vi "Affichage PokaenDex.vi"() -> ()   [LabVIEW 2013]
uses:
  <vilib>/picture/picture.llb/Draw True-Color Pixmap.vi
panel:
  in  "Bouton OK 2":bool
  in  "Port USB en réception":refnum<visa-resource-name>="ASRL1::INSTR"
  out "Cache rouge":picture
  out "Ami 2":bool
  out "2":bool
  out "Image 2D":picture
  out "sign 2":u32
  out "Distance cible 2":string
  out "sign 1":u32
  out "Distance cible 1":string
  out "Cam D détect":bool
  out "2 cam détect":bool
  out "Cam G détect":bool
  in  "2D/3D":bool caption="Booléen 5"
  in  "Booléen":bool
  out "1":bool
  out "Ami":bool
  out "Cache gris":picture
  out "Nom du Pokaenmon":string
  out "Nom du Pokaenmon 2":string
  out "Pokeanmon détécté !":bool
  in  "stop":bool
  out "Image Pokaenmon 2":picture
  out "Image Pokaenmon":picture
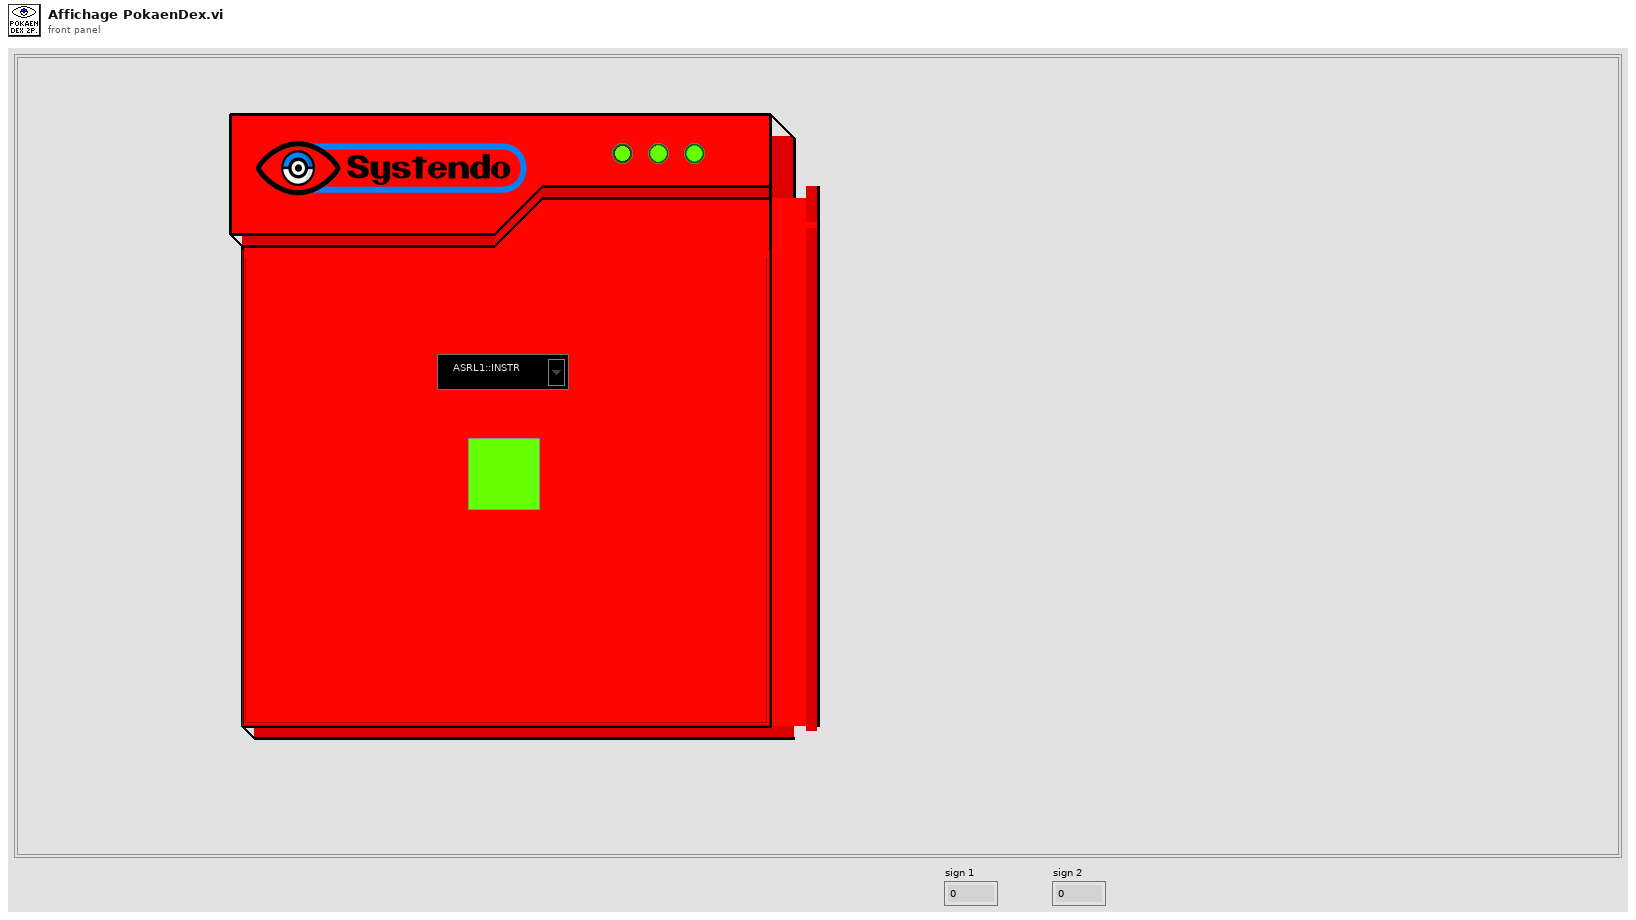
[diagram p1: front panel]
types:
  T1 = cluster{"left":i16, "top":i16, "right":i16, "bottom":i16}
  T2 = cluster{"Pokaenmon détecté":bool, "Signature":u32, "x":dbl, "y ":dbl, "Longueur":dbl, "Hauteur":dbl}
  T3 = cluster{"Données Caméra G":cluster{dbl, dbl, dbl, dbl}, "Données Caméra D":cluster{dbl, dbl, dbl, dbl}}
  T4 = typedef "imagedata.ctl" = cluster{"image type":i32, "image depth":i32, "image":u8[], "mask":u8[], "colors":u32[], "Rectangle":cluster{"left":i16, "top":i16, "right":i16, "bottom":i16}}
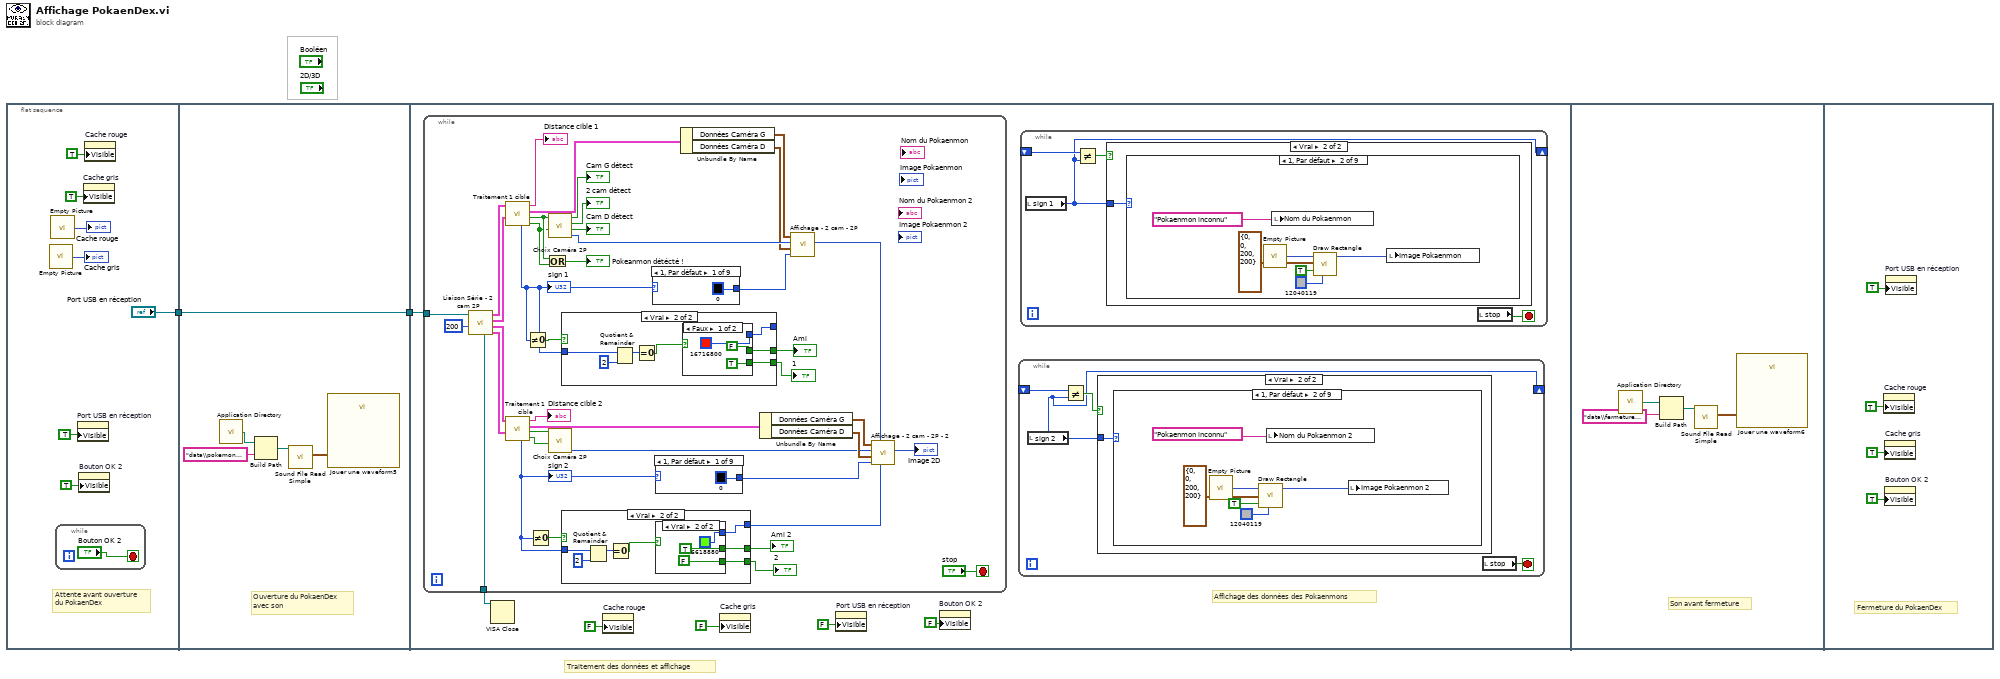
[diagram p0: block diagram]
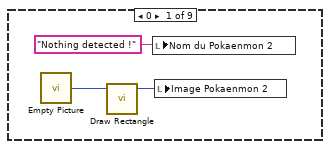
[diagram p3: hidden frame]
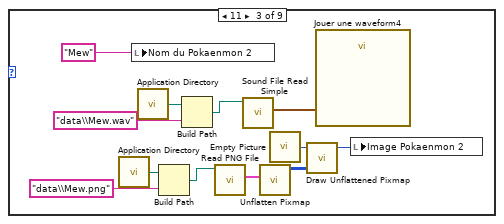
[diagram p4: hidden frame]
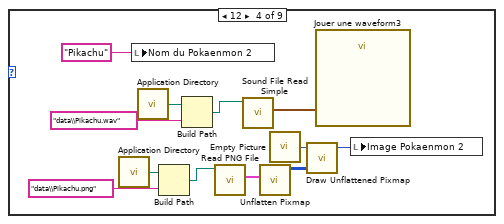
[diagram p5: hidden frame]
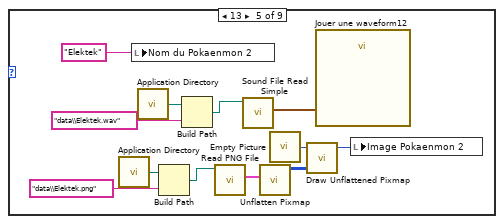
[diagram p6: hidden frame]
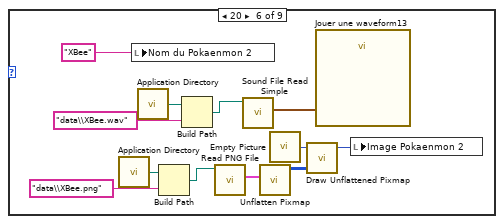
[diagram p7: hidden frame]
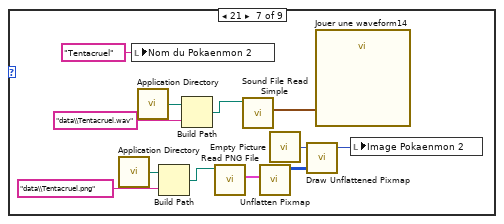
[diagram p8: hidden frame]
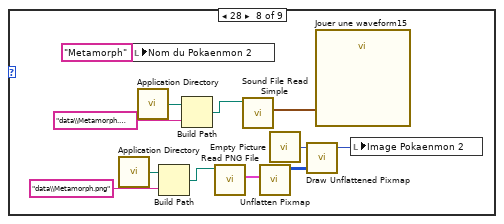
[diagram p9: hidden frame]
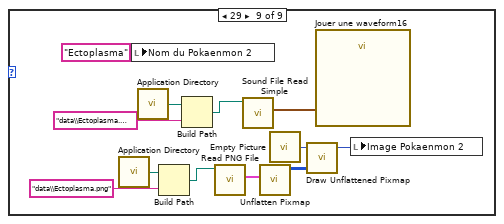
[diagram p10: hidden frame]
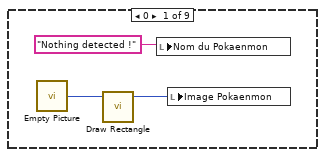
[diagram p12: hidden frame]
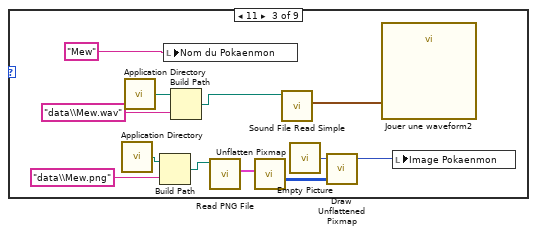
[diagram p13: hidden frame]
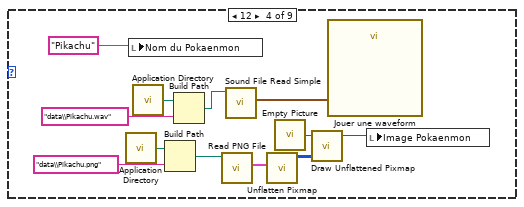
[diagram p14: hidden frame]
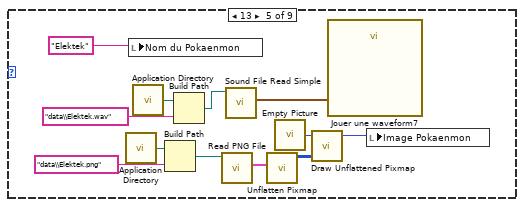
[diagram p15: hidden frame]
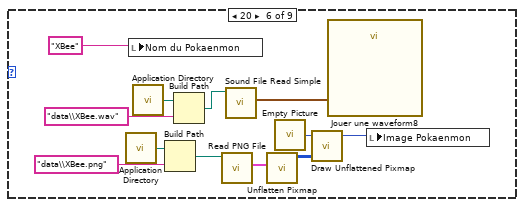
[diagram p16: hidden frame]
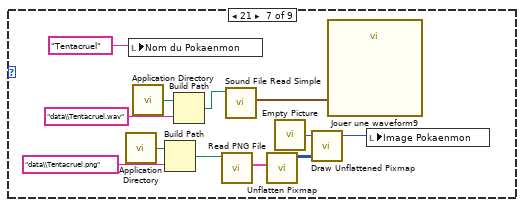
[diagram p17: hidden frame]
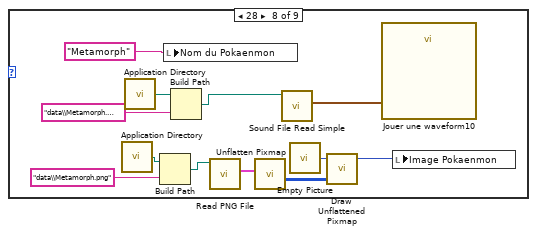
[diagram p18: hidden frame]
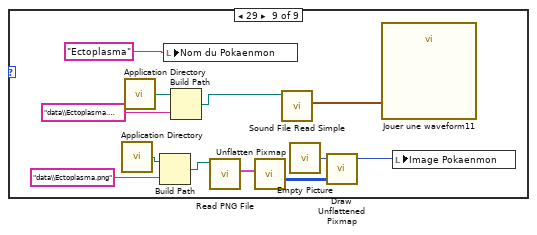
[diagram p19: hidden frame]
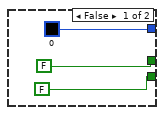
[diagram p20: hidden frame]
diagram:
  # "Traitement des données et affichage"
  n1 = flat-sequence {
    tunnel: ["Port USB en réception"] -> w2
    tunnel: w2 -> [w15]
    tunnel: [w15] -> w1
    tunnel: w1 -> [w20]
    frame #0 {
      # "Attente avant ouverture\ndu PokaenDex"
      n2 = call "Empty Picture"() -> ("empty picture"=→"Cache gris":picture)
      n3 = call "Empty Picture"() -> ("empty picture"=→"Cache rouge":picture)
      n4 = while {
        stop <- "Bouton OK 2" stop-if-true
      }
      n5 = property on="Port USB en réception" class="NomVISA"("Visible"=TRUE) -> ()  [unwired: 2 in, 2 out]
      n6 = property on="Bouton OK 2" class="Bool"("Visible"=TRUE) -> ()  [unwired: 2 in, 2 out]
      n7 = property on="Cache gris" class="Image"("Visible"=TRUE) -> ()  [unwired: 2 in, 2 out]
      n8 = property on="Cache rouge" class="Image"("Visible"=TRUE) -> ()  [unwired: 2 in, 2 out]
    }
    frame #1 {
      # "Ouverture du PokaenDex\navec son"
      n9 = call <vilib>:"Application Directory.vi"() -> ("Application Directory"=w11:path)
      n10 = Build Path(base path=w11, name or relative path="data\\pokemon ouverture.wav") -> (appended path=w12:path)
      n11 = call <vilib>:"Sound File Read Simple.vi"("path"=w12) -> ("data"=w14:waveform(dbl)[])  [unwired: 7 in, 3 out]
      n12 = call "Jouer une waveform5"("Data"=w14) -> ()  [unwired: 18 in, 1 out]
    }
    frame #2 {
      # "Affichage des données des Pokaenmons"
      n13 = while {
        tunnel: w20 -> [w249]
        tunnel: [w248] -> w21
        stop <- "stop" stop-if-true
        n14 = call "Liaison Série - 2 cam 2P.vi"("timeout (ms)"=u32 200 ("timeout (10sec)"), "Port USB en réception"=w249) -> ("Indications pokaenmon D 2"=w238:T2, "Indications pokaenmon G 2"=w239:T2, "Indications pokaenmon D"=w240:T2, "Indications pokaenmon G"=w247:T2, "Nom VISA en sortie"=w248:refnum<visa-resource-name>)  [unwired: 5 in]
        n15 = call "Traitement 1 cible.vi"("Indications Pokaenmon D"=w240, "Indications Pokaenmon G"=w247) -> ("D détect"=w242:bool, "G détect"=w243:bool, "Données caméras"=w246:T3, "Distance"=→"Distance cible 1":string, "Signature"=w222:u32)  [unwired: 5 in]
        "sign 1" <- w222
        n16 = call "Traitement 1 cible.vi"("Indications Pokaenmon D"=w238, "Indications Pokaenmon G"=w239) -> ("D détect"=w229:bool, "G détect"=w230:bool, "Données caméras"=w234:T3, "Distance"=→"Distance cible 2":string, "Signature"=w226:u32)  [unwired: 5 in]
        "sign 2" <- w226
        n17 = Not Equal To 0?(x=w222) -> (x != 0?=w223:bool)
        n18 = Not Equal To 0?(x=w226) -> (x != 0?=w227:bool)
        n19 = Or(x=w243, y=w242) -> (x .or. y?=→"Pokeanmon détécté !":bool)
        n20 = call "Choix Caméra 2P.vi"("Detecté caméra D"=w242, "Detecté caméra G"=w243) -> ("Choix"=w255:u16, "Detecté caméra D"=→"Cam D détect":bool, "Detecté caméra G et D"=→"2 cam détect":bool, "Detecté caméra G"=→"Cam G détect":bool)  [unwired: 6 in]
        n21 = call "Choix Caméra 2P.vi"("Detecté caméra D"=w229, "Detecté caméra G"=w230) -> ("Choix"=w231:u16)  [unwired: 6 in, 3 out]
        n22 = case shown="Vrai" w227 {
          tunnel: w226 -> [_ w288]
          tunnel: [u32 0 ("Couleur rectangle") w287] -> w225
          tunnel: [FALSE w286] -> w219
          tunnel: [FALSE w285] -> w218
          frame False {
          }
          frame True {
            n23 = Quotient & Remainder(x=w288, y=2) -> (x-y*floor(x/y)=w291:u32)  [unwired: 1 out]
            n24 = Equal To 0?(x=w291) -> (x = 0?=w289:bool)
            n25 = case shown="Vrai" w289 {
              tunnel: [u32 16716800 ("Couleur rectangle") u32 6618880 ("Couleur rectangle")] -> w287
              tunnel: [FALSE TRUE] -> w286
              tunnel: [TRUE FALSE] -> w285
              frame False {
              }
              frame True {
              }
            }
          }
        }
        "Ami 2" <- w219
        "2" <- w218
        n26 = case shown="Vrai" w223 {
          tunnel: w222 -> [_ w263]
          tunnel: [u32 0 ("Couleur rectangle") w262] -> _
          tunnel: [FALSE w261] -> w221
          tunnel: [FALSE w260] -> w220
          frame False {
          }
          frame True {
            n27 = Quotient & Remainder(x=w263, y=2) -> (x-y*floor(x/y)=w266:u32)  [unwired: 1 out]
            n28 = Equal To 0?(x=w266) -> (x = 0?=w264:bool)
            n29 = case shown="Faux" w264 {
              tunnel: [u32 16716800 ("Couleur rectangle") u32 6618880 ("Couleur rectangle")] -> w262
              tunnel: [FALSE TRUE] -> w261
              tunnel: [TRUE FALSE] -> w260
              frame False {
              }
              frame True {
              }
            }
          }
        }
        "Ami" <- w221
        "1" <- w220
        n30 = case shown="1, Par défaut" w222 {
          tunnel: [u32 0 ("Couleur rectangle") u32 32639 ("Couleur rectangle") u32 16752871 ("Couleur rectangle") u32 14483200 ("Couleur rectangle") u32 16766208 ("Couleur rectangle") u32 2817023 ("Couleur rectangle") u32 4342527 ("Couleur rectangle") u32 16716454 ("Couleur rectangle") u32 11141359 ("Couleur rectangle")] -> w224
          frame 1, Default {
          }
          frame 2 {
          }
          frame 11 {
          }
          frame 12 {
          }
          frame 13 {
          }
          frame 20 {
          }
          frame 21 {
          }
          frame 29 {
          }
          frame 28 {
          }
        }
        n31 = case shown="1, Par défaut" w226 {
          tunnel: [u32 0 ("Couleur rectangle") u32 32639 ("Couleur rectangle") u32 16752871 ("Couleur rectangle") u32 14483200 ("Couleur rectangle") u32 16766208 ("Couleur rectangle") u32 2817023 ("Couleur rectangle") u32 4342527 ("Couleur rectangle") u32 16716454 ("Couleur rectangle") u32 11141359 ("Couleur rectangle")] -> w235
          frame 1, Default {
          }
          frame 2 {
          }
          frame 11 {
          }
          frame 12 {
          }
          frame 13 {
          }
          frame 20 {
          }
          frame 21 {
          }
          frame 29 {
          }
          frame 28 {
          }
        }
        n32 = Unbundle By Name(w246) -> ("Données Caméra G"=w244:cluster{dbl, dbl, dbl, dbl}, "Données Caméra D"=w245:cluster{dbl, dbl, dbl, dbl})
        n33 = Unbundle By Name(w234) -> ("Données Caméra G"=w233:cluster{dbl, dbl, dbl, dbl}, "Données Caméra D"=w232:cluster{dbl, dbl, dbl, dbl})
        n34 = call "Affichage - 2 cam - 2P.vi"("Couleur rectangle"=w224, "Caméra D"=w245, "Choix cam"=w255, "Caméra G"=w244) -> ("Image 2D"=w236:picture)  [unwired: 7 in]
        n35 = call "Affichage - 2 cam - 2P - 2.vi"("Couleur rectangle 2"=w225, "Image 2D 2"=w236, "Couleur rectangle"=w235, "Caméra D"=w232, "Choix cam"=w231, "Caméra G"=w233) -> ("Image 2D"=→"Image 2D":picture)  [unwired: 5 in]
      }
      n36 = VISA Close(VISA resource name=w21) -> ()  [unwired: 1 in, 1 out]
      n37 = property on="Cache rouge" class="Image"("Visible"=FALSE) -> ()  [unwired: 2 in, 2 out]
      n38 = property on="Cache gris" class="Image"("Visible"=FALSE) -> ()  [unwired: 2 in, 2 out]
      n39 = property on="Port USB en réception" class="NomVISA"("Visible"=FALSE) -> ()  [unwired: 2 in, 2 out]
      n40 = property on="Bouton OK 2" class="Bool"("Visible"=FALSE) -> ()  [unwired: 2 in, 2 out]
      n41 = while {
        shift-right: [w22] -> _
        shift-left: _ -> [w24]
        stop <- w25 stop-if-true
        n42 = local read "sign 2"() -> (w22:u32)
        n43 = Not Equal?(x=w24, y=w22) -> (x != y?=w23:bool)
        n44 = case shown="Vrai" w23 {
          tunnel: w22 -> [_ w26]
          frame False {
          }
          frame True {
            n45 = case shown="1, Par défaut" w26 {
              frame 0 {
                n46 = call "Empty Picture"() -> ("empty picture"=w29:picture)
                n47 = call <vilib>:"Draw Rectangle.vi"("picture"=w29) -> ("new picture"=w28:picture)  [unwired: 8 in]
                n48 = local write "Nom du Pokaenmon 2"("Nothing detected !") -> ()
                n49 = local write "Image Pokaenmon 2"(w28) -> ()
              }
              frame 1, Default {
                n50 = call "Empty Picture"() -> ("empty picture"=w34:picture)
                n51 = call <vilib>:"Draw Rectangle.vi"("picture"=w34, "rect"=T1 {"left"=0, "top"=0, "right"=200, "bottom"=200}, "fill?(F)"=TRUE, "color(black)"=u32 12040119) -> ("new picture"=w33:picture)  [unwired: 5 in]
                n52 = local write "Nom du Pokaenmon 2"("Pokaenmon inconnu") -> ()
                n53 = local write "Image Pokaenmon 2"(w33) -> ()
              }
              frame 11 {
                n54 = call <vilib>:"Application Directory.vi"() -> ("Application Directory"=w36:path)
                n55 = local write "Nom du Pokaenmon 2"("Mew") -> ()
                n56 = call <vilib>:"Application Directory.vi"() -> ("Application Directory"=w37:path)
                n57 = Build Path(base path=w36, name or relative path="data\\Mew.png") -> (appended path=w38:path)
                n58 = Build Path(base path=w37, name or relative path="data\\Mew.wav") -> (appended path=w39:path)
                n59 = call <vilib>:"Read PNG File.vi"("path to PNG file"=w38) -> ("image data"=w46:T4)  [unwired: 8 in, 2 out]
                n60 = call <vilib>:"Sound File Read Simple.vi"("path"=w39) -> ("data"=w44:waveform(dbl)[])  [unwired: 7 in, 3 out]
                n61 = call <vilib>:"Unflatten Pixmap.vi"("image data"=w46) -> ("24-bit pixmap"=w45:u32[][])  [unwired: 4 in, 6 out]
                n62 = call "Empty Picture"() -> ("empty picture"=w47:picture)
                n63 = call-poly <vilib>:"Draw Unflattened Pixmap.vi"("picture"=w47, "data (RGB format)"=w45) -> ("new picture"=w43:picture)  [unwired: 7 in]
                n64 = call "Jouer une waveform4"("Data"=w44) -> ()  [unwired: 18 in, 1 out]
                n65 = local write "Image Pokaenmon 2"(w43) -> ()
              }
              frame 12 {
                n66 = call <vilib>:"Application Directory.vi"() -> ("Application Directory"=w48:path)
                n67 = local write "Nom du Pokaenmon 2"("Pikachu") -> ()
                n68 = call <vilib>:"Application Directory.vi"() -> ("Application Directory"=w49:path)
                n69 = Build Path(base path=w48, name or relative path="data\\Pikachu.png") -> (appended path=w50:path)
                n70 = Build Path(base path=w49, name or relative path="data\\Pikachu.wav") -> (appended path=w51:path)
                n71 = call <vilib>:"Read PNG File.vi"("path to PNG file"=w50) -> ("image data"=w58:T4)  [unwired: 8 in, 2 out]
                n72 = call <vilib>:"Sound File Read Simple.vi"("path"=w51) -> ("data"=w56:waveform(dbl)[])  [unwired: 7 in, 3 out]
                n73 = call <vilib>:"Unflatten Pixmap.vi"("image data"=w58) -> ("24-bit pixmap"=w57:u32[][])  [unwired: 4 in, 6 out]
                n74 = call "Empty Picture"() -> ("empty picture"=w59:picture)
                n75 = call-poly <vilib>:"Draw Unflattened Pixmap.vi"("picture"=w59, "data (RGB format)"=w57) -> ("new picture"=w55:picture)  [unwired: 7 in]
                n76 = call "Jouer une waveform3"("Data"=w56) -> ()  [unwired: 18 in, 1 out]
                n77 = local write "Image Pokaenmon 2"(w55) -> ()
              }
              frame 13 {
                n78 = call <vilib>:"Application Directory.vi"() -> ("Application Directory"=w60:path)
                n79 = local write "Nom du Pokaenmon 2"("Elektek") -> ()
                n80 = call <vilib>:"Application Directory.vi"() -> ("Application Directory"=w61:path)
                n81 = Build Path(base path=w60, name or relative path="data\\Elektek.png") -> (appended path=w62:path)
                n82 = Build Path(base path=w61, name or relative path="data\\Elektek.wav") -> (appended path=w63:path)
                n83 = call <vilib>:"Read PNG File.vi"("path to PNG file"=w62) -> ("image data"=w70:T4)  [unwired: 8 in, 2 out]
                n84 = call <vilib>:"Sound File Read Simple.vi"("path"=w63) -> ("data"=w68:waveform(dbl)[])  [unwired: 7 in, 3 out]
                n85 = call <vilib>:"Unflatten Pixmap.vi"("image data"=w70) -> ("24-bit pixmap"=w69:u32[][])  [unwired: 4 in, 6 out]
                n86 = call "Empty Picture"() -> ("empty picture"=w71:picture)
                n87 = call-poly <vilib>:"Draw Unflattened Pixmap.vi"("picture"=w71, "data (RGB format)"=w69) -> ("new picture"=w67:picture)  [unwired: 7 in]
                n88 = call "Jouer une waveform12"("Data"=w68) -> ()  [unwired: 18 in, 1 out]
                n89 = local write "Image Pokaenmon 2"(w67) -> ()
              }
              frame 20 {
                n90 = call <vilib>:"Application Directory.vi"() -> ("Application Directory"=w72:path)
                n91 = local write "Nom du Pokaenmon 2"("XBee") -> ()
                n92 = call <vilib>:"Application Directory.vi"() -> ("Application Directory"=w73:path)
                n93 = Build Path(base path=w72, name or relative path="data\\XBee.png") -> (appended path=w74:path)
                n94 = Build Path(base path=w73, name or relative path="data\\XBee.wav") -> (appended path=w75:path)
                n95 = call <vilib>:"Read PNG File.vi"("path to PNG file"=w74) -> ("image data"=w82:T4)  [unwired: 8 in, 2 out]
                n96 = call <vilib>:"Sound File Read Simple.vi"("path"=w75) -> ("data"=w80:waveform(dbl)[])  [unwired: 7 in, 3 out]
                n97 = call <vilib>:"Unflatten Pixmap.vi"("image data"=w82) -> ("24-bit pixmap"=w81:u32[][])  [unwired: 4 in, 6 out]
                n98 = call "Empty Picture"() -> ("empty picture"=w83:picture)
                n99 = call-poly <vilib>:"Draw Unflattened Pixmap.vi"("picture"=w83, "data (RGB format)"=w81) -> ("new picture"=w79:picture)  [unwired: 7 in]
                n100 = call "Jouer une waveform13"("Data"=w80) -> ()  [unwired: 18 in, 1 out]
                n101 = local write "Image Pokaenmon 2"(w79) -> ()
              }
              frame 21 {
                n102 = call <vilib>:"Application Directory.vi"() -> ("Application Directory"=w84:path)
                n103 = local write "Nom du Pokaenmon 2"("Tentacruel") -> ()
                n104 = call <vilib>:"Application Directory.vi"() -> ("Application Directory"=w85:path)
                n105 = Build Path(base path=w84, name or relative path="data\\Tentacruel.png") -> (appended path=w86:path)
                n106 = Build Path(base path=w85, name or relative path="data\\Tentacruel.wav") -> (appended path=w87:path)
                n107 = call <vilib>:"Read PNG File.vi"("path to PNG file"=w86) -> ("image data"=w94:T4)  [unwired: 8 in, 2 out]
                n108 = call <vilib>:"Sound File Read Simple.vi"("path"=w87) -> ("data"=w92:waveform(dbl)[])  [unwired: 7 in, 3 out]
                n109 = call <vilib>:"Unflatten Pixmap.vi"("image data"=w94) -> ("24-bit pixmap"=w93:u32[][])  [unwired: 4 in, 6 out]
                n110 = call "Empty Picture"() -> ("empty picture"=w95:picture)
                n111 = call-poly <vilib>:"Draw Unflattened Pixmap.vi"("picture"=w95, "data (RGB format)"=w93) -> ("new picture"=w91:picture)  [unwired: 7 in]
                n112 = call "Jouer une waveform14"("Data"=w92) -> ()  [unwired: 18 in, 1 out]
                n113 = local write "Image Pokaenmon 2"(w91) -> ()
              }
              frame 28 {
                n114 = call <vilib>:"Application Directory.vi"() -> ("Application Directory"=w96:path)
                n115 = local write "Nom du Pokaenmon 2"("Metamorph") -> ()
                n116 = call <vilib>:"Application Directory.vi"() -> ("Application Directory"=w97:path)
                n117 = Build Path(base path=w96, name or relative path="data\\Metamorph.png") -> (appended path=w98:path)
                n118 = Build Path(base path=w97, name or relative path="data\\Metamorph.wav") -> (appended path=w99:path)
                n119 = call <vilib>:"Read PNG File.vi"("path to PNG file"=w98) -> ("image data"=w106:T4)  [unwired: 8 in, 2 out]
                n120 = call <vilib>:"Sound File Read Simple.vi"("path"=w99) -> ("data"=w104:waveform(dbl)[])  [unwired: 7 in, 3 out]
                n121 = call <vilib>:"Unflatten Pixmap.vi"("image data"=w106) -> ("24-bit pixmap"=w105:u32[][])  [unwired: 4 in, 6 out]
                n122 = call "Empty Picture"() -> ("empty picture"=w107:picture)
                n123 = call-poly <vilib>:"Draw Unflattened Pixmap.vi"("picture"=w107, "data (RGB format)"=w105) -> ("new picture"=w103:picture)  [unwired: 7 in]
                n124 = call "Jouer une waveform15"("Data"=w104) -> ()  [unwired: 18 in, 1 out]
                n125 = local write "Image Pokaenmon 2"(w103) -> ()
              }
              frame 29 {
                n126 = call <vilib>:"Application Directory.vi"() -> ("Application Directory"=w108:path)
                n127 = local write "Nom du Pokaenmon 2"("Ectoplasma") -> ()
                n128 = call <vilib>:"Application Directory.vi"() -> ("Application Directory"=w109:path)
                n129 = Build Path(base path=w108, name or relative path="data\\Ectoplasma.png") -> (appended path=w110:path)
                n130 = Build Path(base path=w109, name or relative path="data\\Ectoplasma.wav") -> (appended path=w111:path)
                n131 = call <vilib>:"Read PNG File.vi"("path to PNG file"=w110) -> ("image data"=w118:T4)  [unwired: 8 in, 2 out]
                n132 = call <vilib>:"Sound File Read Simple.vi"("path"=w111) -> ("data"=w116:waveform(dbl)[])  [unwired: 7 in, 3 out]
                n133 = call <vilib>:"Unflatten Pixmap.vi"("image data"=w118) -> ("24-bit pixmap"=w117:u32[][])  [unwired: 4 in, 6 out]
                n134 = call "Empty Picture"() -> ("empty picture"=w119:picture)
                n135 = call-poly <vilib>:"Draw Unflattened Pixmap.vi"("picture"=w119, "data (RGB format)"=w117) -> ("new picture"=w115:picture)  [unwired: 7 in]
                n136 = call "Jouer une waveform16"("Data"=w116) -> ()  [unwired: 18 in, 1 out]
                n137 = local write "Image Pokaenmon 2"(w115) -> ()
              }
            }
          }
        }
        n138 = local read "stop"() -> (w25:bool)
      }
      n139 = while {
        shift-right: [w120] -> _
        shift-left: _ -> [w122]
        stop <- w123 stop-if-true
        n140 = local read "sign 1"() -> (w120:u32)
        n141 = Not Equal?(x=w122, y=w120) -> (x != y?=w121:bool)
        n142 = case shown="Vrai" w121 {
          tunnel: w120 -> [_ w124]
          frame False {
          }
          frame True {
            n143 = case shown="1, Par défaut" w124 {
              frame 0 {
                n144 = call "Empty Picture"() -> ("empty picture"=w127:picture)
                n145 = call <vilib>:"Draw Rectangle.vi"("picture"=w127) -> ("new picture"=w125:picture)  [unwired: 8 in]
                n146 = local write "Nom du Pokaenmon"("Nothing detected !") -> ()
                n147 = local write "Image Pokaenmon"(w125) -> ()
              }
              frame 1, Default {
                n148 = call "Empty Picture"() -> ("empty picture"=w132:picture)
                n149 = local write "Nom du Pokaenmon"("Pokaenmon inconnu") -> ()
                n150 = call <vilib>:"Draw Rectangle.vi"("picture"=w132, "rect"=T1 {"left"=0, "top"=0, "right"=200, "bottom"=200}, "fill?(F)"=TRUE, "color(black)"=u32 12040119) -> ("new picture"=w131:picture)  [unwired: 5 in]
                n151 = local write "Image Pokaenmon"(w131) -> ()
              }
              frame 11 {
                n152 = call <vilib>:"Application Directory.vi"() -> ("Application Directory"=w134:path)
                n153 = call <vilib>:"Application Directory.vi"() -> ("Application Directory"=w135:path)
                n154 = Build Path(base path=w134, name or relative path="data\\Mew.png") -> (appended path=w138:path)
                n155 = local write "Nom du Pokaenmon"("Mew") -> ()
                n156 = Build Path(base path=w135, name or relative path="data\\Mew.wav") -> (appended path=w136:path)
                n157 = call <vilib>:"Read PNG File.vi"("path to PNG file"=w138) -> ("image data"=w144:T4)  [unwired: 8 in, 2 out]
                n158 = call <vilib>:"Unflatten Pixmap.vi"("image data"=w144) -> ("24-bit pixmap"=w143:u32[][])  [unwired: 4 in, 6 out]
                n159 = call <vilib>:"Sound File Read Simple.vi"("path"=w136) -> ("data"=w140:waveform(dbl)[])  [unwired: 7 in, 3 out]
                n160 = call "Empty Picture"() -> ("empty picture"=w145:picture)
                n161 = call-poly <vilib>:"Draw Unflattened Pixmap.vi"("picture"=w145, "data (RGB format)"=w143) -> ("new picture"=w141:picture)  [unwired: 7 in]
                n162 = call "Jouer une waveform2"("Data"=w140) -> ()  [unwired: 18 in, 1 out]
                n163 = local write "Image Pokaenmon"(w141) -> ()
              }
              frame 12 {
                n164 = call <vilib>:"Application Directory.vi"() -> ("Application Directory"=w146:path)
                n165 = local write "Nom du Pokaenmon"("Pikachu") -> ()
                n166 = call <vilib>:"Application Directory.vi"() -> ("Application Directory"=w147:path)
                n167 = Build Path(base path=w146, name or relative path="data\\Pikachu.png") -> (appended path=w148:path)
                n168 = Build Path(base path=w147, name or relative path="data\\Pikachu.wav") -> (appended path=w150:path)
                n169 = call <vilib>:"Read PNG File.vi"("path to PNG file"=w148) -> ("image data"=w156:T4)  [unwired: 8 in, 2 out]
                n170 = call <vilib>:"Sound File Read Simple.vi"("path"=w150) -> ("data"=w152:waveform(dbl)[])  [unwired: 7 in, 3 out]
                n171 = call <vilib>:"Unflatten Pixmap.vi"("image data"=w156) -> ("24-bit pixmap"=w155:u32[][])  [unwired: 4 in, 6 out]
                n172 = call "Empty Picture"() -> ("empty picture"=w157:picture)
                n173 = call-poly <vilib>:"Draw Unflattened Pixmap.vi"("picture"=w157, "data (RGB format)"=w155) -> ("new picture"=w153:picture)  [unwired: 7 in]
                n174 = call "Jouer une waveform"("Data"=w152) -> ()  [unwired: 18 in, 1 out]
                n175 = local write "Image Pokaenmon"(w153) -> ()
              }
              frame 13 {
                n176 = call <vilib>:"Application Directory.vi"() -> ("Application Directory"=w158:path)
                n177 = local write "Nom du Pokaenmon"("Elektek") -> ()
                n178 = call <vilib>:"Application Directory.vi"() -> ("Application Directory"=w159:path)
                n179 = Build Path(base path=w158, name or relative path="data\\Elektek.png") -> (appended path=w160:path)
                n180 = Build Path(base path=w159, name or relative path="data\\Elektek.wav") -> (appended path=w162:path)
                n181 = call <vilib>:"Read PNG File.vi"("path to PNG file"=w160) -> ("image data"=w168:T4)  [unwired: 8 in, 2 out]
                n182 = call <vilib>:"Sound File Read Simple.vi"("path"=w162) -> ("data"=w164:waveform(dbl)[])  [unwired: 7 in, 3 out]
                n183 = call <vilib>:"Unflatten Pixmap.vi"("image data"=w168) -> ("24-bit pixmap"=w167:u32[][])  [unwired: 4 in, 6 out]
                n184 = call "Empty Picture"() -> ("empty picture"=w169:picture)
                n185 = call-poly <vilib>:"Draw Unflattened Pixmap.vi"("picture"=w169, "data (RGB format)"=w167) -> ("new picture"=w165:picture)  [unwired: 7 in]
                n186 = call "Jouer une waveform7"("Data"=w164) -> ()  [unwired: 18 in, 1 out]
                n187 = local write "Image Pokaenmon"(w165) -> ()
              }
              frame 20 {
                n188 = call <vilib>:"Application Directory.vi"() -> ("Application Directory"=w170:path)
                n189 = local write "Nom du Pokaenmon"("XBee") -> ()
                n190 = call <vilib>:"Application Directory.vi"() -> ("Application Directory"=w171:path)
                n191 = Build Path(base path=w170, name or relative path="data\\XBee.png") -> (appended path=w172:path)
                n192 = Build Path(base path=w171, name or relative path="data\\XBee.wav") -> (appended path=w174:path)
                n193 = call <vilib>:"Read PNG File.vi"("path to PNG file"=w172) -> ("image data"=w180:T4)  [unwired: 8 in, 2 out]
                n194 = call <vilib>:"Sound File Read Simple.vi"("path"=w174) -> ("data"=w176:waveform(dbl)[])  [unwired: 7 in, 3 out]
                n195 = call <vilib>:"Unflatten Pixmap.vi"("image data"=w180) -> ("24-bit pixmap"=w179:u32[][])  [unwired: 4 in, 6 out]
                n196 = call "Empty Picture"() -> ("empty picture"=w181:picture)
                n197 = call-poly <vilib>:"Draw Unflattened Pixmap.vi"("picture"=w181, "data (RGB format)"=w179) -> ("new picture"=w177:picture)  [unwired: 7 in]
                n198 = call "Jouer une waveform8"("Data"=w176) -> ()  [unwired: 18 in, 1 out]
                n199 = local write "Image Pokaenmon"(w177) -> ()
              }
              frame 21 {
                n200 = call <vilib>:"Application Directory.vi"() -> ("Application Directory"=w182:path)
                n201 = local write "Nom du Pokaenmon"("Tentacruel") -> ()
                n202 = call <vilib>:"Application Directory.vi"() -> ("Application Directory"=w183:path)
                n203 = Build Path(base path=w182, name or relative path="data\\Tentacruel.png") -> (appended path=w184:path)
                n204 = Build Path(base path=w183, name or relative path="data\\Tentacruel.wav") -> (appended path=w186:path)
                n205 = call <vilib>:"Read PNG File.vi"("path to PNG file"=w184) -> ("image data"=w192:T4)  [unwired: 8 in, 2 out]
                n206 = call <vilib>:"Sound File Read Simple.vi"("path"=w186) -> ("data"=w188:waveform(dbl)[])  [unwired: 7 in, 3 out]
                n207 = call <vilib>:"Unflatten Pixmap.vi"("image data"=w192) -> ("24-bit pixmap"=w191:u32[][])  [unwired: 4 in, 6 out]
                n208 = call "Empty Picture"() -> ("empty picture"=w193:picture)
                n209 = call-poly <vilib>:"Draw Unflattened Pixmap.vi"("picture"=w193, "data (RGB format)"=w191) -> ("new picture"=w189:picture)  [unwired: 7 in]
                n210 = call "Jouer une waveform9"("Data"=w188) -> ()  [unwired: 18 in, 1 out]
                n211 = local write "Image Pokaenmon"(w189) -> ()
              }
              frame 28 {
                n212 = call <vilib>:"Application Directory.vi"() -> ("Application Directory"=w194:path)
                n213 = call <vilib>:"Application Directory.vi"() -> ("Application Directory"=w195:path)
                n214 = Build Path(base path=w194, name or relative path="data\\Metamorph.png") -> (appended path=w198:path)
                n215 = local write "Nom du Pokaenmon"("Metamorph") -> ()
                n216 = Build Path(base path=w195, name or relative path="data\\Metamorph.wav") -> (appended path=w196:path)
                n217 = call <vilib>:"Read PNG File.vi"("path to PNG file"=w198) -> ("image data"=w204:T4)  [unwired: 8 in, 2 out]
                n218 = call <vilib>:"Unflatten Pixmap.vi"("image data"=w204) -> ("24-bit pixmap"=w203:u32[][])  [unwired: 4 in, 6 out]
                n219 = call <vilib>:"Sound File Read Simple.vi"("path"=w196) -> ("data"=w200:waveform(dbl)[])  [unwired: 7 in, 3 out]
                n220 = call "Empty Picture"() -> ("empty picture"=w205:picture)
                n221 = call-poly <vilib>:"Draw Unflattened Pixmap.vi"("picture"=w205, "data (RGB format)"=w203) -> ("new picture"=w201:picture)  [unwired: 7 in]
                n222 = call "Jouer une waveform10"("Data"=w200) -> ()  [unwired: 18 in, 1 out]
                n223 = local write "Image Pokaenmon"(w201) -> ()
              }
              frame 29 {
                n224 = call <vilib>:"Application Directory.vi"() -> ("Application Directory"=w206:path)
                n225 = call <vilib>:"Application Directory.vi"() -> ("Application Directory"=w207:path)
                n226 = Build Path(base path=w206, name or relative path="data\\Ectoplasma.png") -> (appended path=w210:path)
                n227 = local write "Nom du Pokaenmon"("Ectoplasma") -> ()
                n228 = Build Path(base path=w207, name or relative path="data\\Ectoplasma.wav") -> (appended path=w208:path)
                n229 = call <vilib>:"Read PNG File.vi"("path to PNG file"=w210) -> ("image data"=w216:T4)  [unwired: 8 in, 2 out]
                n230 = call <vilib>:"Unflatten Pixmap.vi"("image data"=w216) -> ("24-bit pixmap"=w215:u32[][])  [unwired: 4 in, 6 out]
                n231 = call <vilib>:"Sound File Read Simple.vi"("path"=w208) -> ("data"=w212:waveform(dbl)[])  [unwired: 7 in, 3 out]
                n232 = call "Empty Picture"() -> ("empty picture"=w217:picture)
                n233 = call-poly <vilib>:"Draw Unflattened Pixmap.vi"("picture"=w217, "data (RGB format)"=w215) -> ("new picture"=w213:picture)  [unwired: 7 in]
                n234 = call "Jouer une waveform11"("Data"=w212) -> ()  [unwired: 18 in, 1 out]
                n235 = local write "Image Pokaenmon"(w213) -> ()
              }
            }
          }
        }
        n236 = local read "stop"() -> (w123:bool)
      }
    }
    frame #3 {
      # "Son avant fermeture"
      n237 = call <vilib>:"Application Directory.vi"() -> ("Application Directory"=w307:path)
      n238 = Build Path(base path=w307, name or relative path="data\\fermeture pokedex.wav") -> (appended path=w308:path)
      n239 = call <vilib>:"Sound File Read Simple.vi"("path"=w308) -> ("data"=w310:waveform(dbl)[])  [unwired: 7 in, 3 out]
      n240 = call "Jouer une waveform6"("Data"=w310) -> ()  [unwired: 18 in, 1 out]
    }
    frame #4 {
      # "Fermeture du PokaenDex"
      n241 = property on="Cache rouge" class="Image"("Visible"=TRUE) -> ()  [unwired: 2 in, 2 out]
      n242 = property on="Cache gris" class="Image"("Visible"=TRUE) -> ()  [unwired: 2 in, 2 out]
      n243 = property on="Bouton OK 2" class="Bool"("Visible"=TRUE) -> ()  [unwired: 2 in, 2 out]
      n244 = property on="Port USB en réception" class="NomVISA"("Visible"=TRUE) -> ()  [unwired: 2 in, 2 out]
    }
  }
